vi "Test Sync SMO.vi"() -> ()   [LabVIEW 2019, in "DAQmx.lvclass"]
uses:
  DAQmx.lvclass
  typedefs/DAQmx.Status--enum.ctl
  typedefs/DAQmx.Commands--enum.ctl
  typedefs/DAQ.Config.Timing.Sampling--Cluster.ctl
  typedefs/DAQ.Config.AO--Cluster--Array.ctl
  typedefs/DAQ.Config.AO--Cluster.ctl
  typedefs/DAQ.Config.AO.Range--enum.ctl
  typedefs/DAQ.Config.Device Type--enum.ctl
  typedefs/DAQ.Config.AI--Cluster--Array.ctl
  typedefs/DAQ.Config.AI--Cluster.ctl
  typedefs/DAQ.Config.AI.Coupling--enum.ctl
  typedefs/DAQ.Config.AI.Range--enum.ctl
  C:/Program Files/National Instruments/LabVIEW 2019/vi.lib/JKI/JKI SMO/SMO/SMO.lvclass
  <vilib>/JKI/JKI SMO/SMO/SMO.lvclass/SMO.ctl
  <vilib>/JKI/JKI SMO/SMO/Typedefs/SMOState --Enum.ctl
  typedefs/DAQ.Config.Timing--Cluster.ctl
  DAQmx.lvclass/DAQmx.ctl
  6507ff78-a65c-40b2-afe2-716dbe4badb2.vi
  <vilib>/JKI/JKI SMO/SMO/Private/ReftoDVR--SMO.vi
  <vilib>/JKI/JKI SMO/SMO/SMO.lvclass
panel:
  out "delimited string":string
  out "Generator create":i32=5
  out "Generator 'timeout'":i32=729
  out "Generator":i32=733
  out "Waveform Chart":i32(graph)
  out "Waveform Graph":waveform(dbl)[](graph)
  in  "AIconfig":T1=[{"Channels"="PXI1Slot3/ai0", "Coupling"=10050, "Range"=enum."±0.316", "input terminal configuration"=-1, "Type"=enum."PXI-446x"}, {"Channels"="PXI1Slot3/ai1", "Coupling"=10050, "Range"=enum."±0.316", "input terminal configuration"=-1, "Type"=enum."PXI-446x"}, {"Channels"="PXI1Slot5/ai0", "Coupling"=10050, "Range"=enum."±0.316", "input terminal configuration"=-1, "Type"=enum."PXI-446x"}, {"Channels"="PXI1Slot5/ai1", "Coupling"=10050, "Range"=enum."±0.316", "input terminal configuration"=-1, "Type"=enum."PXI-446x"}, {"Channels"="PXI1Slot6/ai0", "Coupling"=10050, "Range"=enum."±0.316", "input terminal configuration"=-1, "Type"=enum."PXI-446x"}, {"Channels"="PXI1Slot6/ai1", "Coupling"=10050, "Range"=enum."±0.316", "input terminal configuration"=-1, "Type"=enum."PXI-446x"}, {"Channels"="PXI1Slot7/ai0", "Coupling"=10050, "Range"=enum."±0.316", "input terminal configuration"=-1, "Type"=enum."PXI-446x"}, {"Channels"="PXI1Slot7/ai1", "Coupling"=10050, "Range"=enum."±0.316", "input terminal configuration"=-1, "Type"=enum."PXI-446x"}, {"Channels"="PXI1Slot8/ai0", "Coupling"=10050, "Range"=enum."±0.316", "input terminal configuration"=-1, "Type"=enum."PXI-446x"}, {"Channels"="PXI1Slot8/ai1", "Coupling"=10050, "Range"=enum."±0.316", "input terminal configuration"=-1, "Type"=enum."PXI-446x"}] {"input terminal configuration" items=[""=-1, "Differential"=10106, "Pseudodifferential"=12529]; "Coupling" items=[""=0, "AC"=10045, "DC"=10050, "GND"=10066]}
  in  "AOconfig":T6=[{"Channels"="PXI1Slot3/ao0", "Range"=enum."±0.1", "output terminal configuration"=-1, "Type"=enum."PXI-446x"}, {"Channels"="PXI1Slot3/ao1", "Range"=enum."±0.1", "output terminal configuration"=-1, "Type"=enum."PXI-446x"}, {"Channels"="PXI1Slot5/ao0", "Range"=enum."±0.1", "output terminal configuration"=-1, "Type"=enum."PXI-446x"}, {"Channels"="PXI1Slot5/ao1", "Range"=enum."±0.1", "output terminal configuration"=-1, "Type"=enum."PXI-446x"}, {"Channels"="PXI1Slot6/ao0", "Range"=enum."±0.1", "output terminal configuration"=-1, "Type"=enum."PXI-446x"}, {"Channels"="PXI1Slot6/ao1", "Range"=enum."±0.1", "output terminal configuration"=-1, "Type"=enum."PXI-446x"}, {"Channels"="PXI1Slot7/ao0", "Range"=enum."±0.1", "output terminal configuration"=-1, "Type"=enum."PXI-446x"}, {"Channels"="PXI1Slot7/ao1", "Range"=enum."±0.1", "output terminal configuration"=-1, "Type"=enum."PXI-446x"}, {"Channels"="PXI1Slot8/ao0", "Range"=enum."±0.1", "output terminal configuration"=-1, "Type"=enum."PXI-446x"}, {"Channels"="PXI1Slot8/ao1", "Range"=enum."±0.1", "output terminal configuration"=-1, "Type"=enum."PXI-446x"}] {"output terminal configuration" items=[""=-1, "Differential"=10106, "Pseudodifferential"=12529]}
  in  "setAIconfig":bool
  in  "setAOconfig":bool
  in  "setTiming":bool
  in  "Sampling":T9={"Fs"=1000.0, "#s"=128} {"Fs" format="%#_13g"}
  in  "setState":bool
  in  "State":T10=enum."auto"
  out "Status":T11
  out "error out":errorcluster
  # "Close Panel to stop the SMO\n(press the \"X\")"
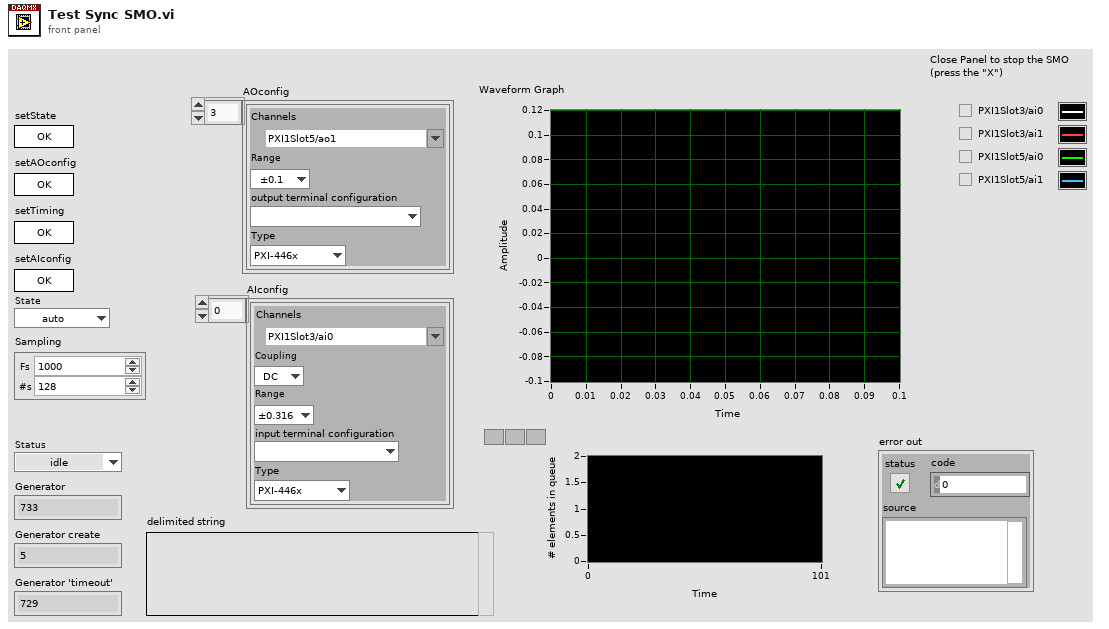
[diagram p1: front panel]
types:
  T1 = typedef "DAQmx.lvclass/DAQ.Config.AI--Cluster--Array.ctl" = T2[]
  T2 = typedef "DAQmx.lvclass/DAQ.Config.AI--Cluster.ctl" = cluster{"Channels":tag, "Coupling":T3, "Range":T4, "input terminal configuration":i32, "Type":T5}
  T3 = typedef "DAQmx.lvclass/DAQ.Config.AI.Coupling--enum.ctl" = u16
  T4 = typedef "DAQmx.lvclass/DAQ.Config.AI.Range--enum.ctl" = enum16{"±0.316", "±1.00", "±3.16", "±10.0", "±31.6", "±42.4", ""}
  T5 = typedef "DAQmx.lvclass/DAQ.Config.Device Type--enum.ctl" = enum16{"None", "USB-4431", "PXI-446x"}
  T6 = typedef "DAQmx.lvclass/DAQ.Config.AO--Cluster--Array.ctl" = T7[]
  T7 = typedef "DAQmx.lvclass/DAQ.Config.AO--Cluster.ctl" = cluster{"Channels":tag, "Range":T8, "output terminal configuration":i32, "Type":T5}
  T8 = typedef "DAQmx.lvclass/DAQ.Config.AO.Range--enum.ctl" = enum16{"±0.1", "±1.0", "±3.5", "±10.0", ""}
  T9 = typedef "DAQmx.lvclass/DAQ.Config.Timing.Sampling--Cluster.ctl" = cluster{"Fs":dbl, "#s":i32}
  T10 = typedef "DAQmx.lvclass/DAQmx.Commands--enum.ctl" = enum16{"idle", "start", "stop", "calibrate", "auto", "exit"}
  T11 = typedef "DAQmx.lvclass/DAQmx.Status--enum.ctl" = enum16{"idle", "calibrating", "configuring", "creating", "created", "starting", "started", "stopping", "stopped", "clearing", "error"}
  T12 = typedef "SMO.lvclass/Public Events.ctl" = cluster{"Error":refnum<user-event>, "State":refnum<user-event>, "Reserve State":refnum<user-event>}
  T13 = typedef "DAQmx.lvclass/PublicEvents--Cluster.ctl" = cluster{"Status":refnum<user-event>, "Devices":refnum<user-event>, "Calibration":refnum<user-event>, "Sampling":refnum<user-event>, "AOconfig":refnum<user-event>, "AIconfig":refnum<user-event>, "Waveforms":refnum<user-event>}
  T14 = cluster{"Event Registration Refnum":refnum<event-registration>}
  T15 = typedef "SMO.lvclass/SMOState --Enum.ctl" = enum16{"unknown", "Created", "Started", "Stopped"}
  T16 = typedef "DAQmx.lvclass/DAQ.Config.Timing--Cluster.ctl" = cluster{"Sampling":T9, "Fs_Out":dbl}
  T17 = typedef "DAQmx.lvclass/DeviceInfo--Cluster.ctl" = cluster{"DeviceName":string, "DevIsSimulated":bool, "DeviceSerialNumber":string, "ProductType":string, "ProductCategory":i32, "ProductNumber":u32, "ChassisNumber":u32, "SlotNumber":u32, "ChassisName":string, "ChassisSerialNumber":string, "DevTemp":dbl, "SelfCal.LastDate/Time":string, "SelfCal.LastTemp":dbl, "calibration due?":bool}
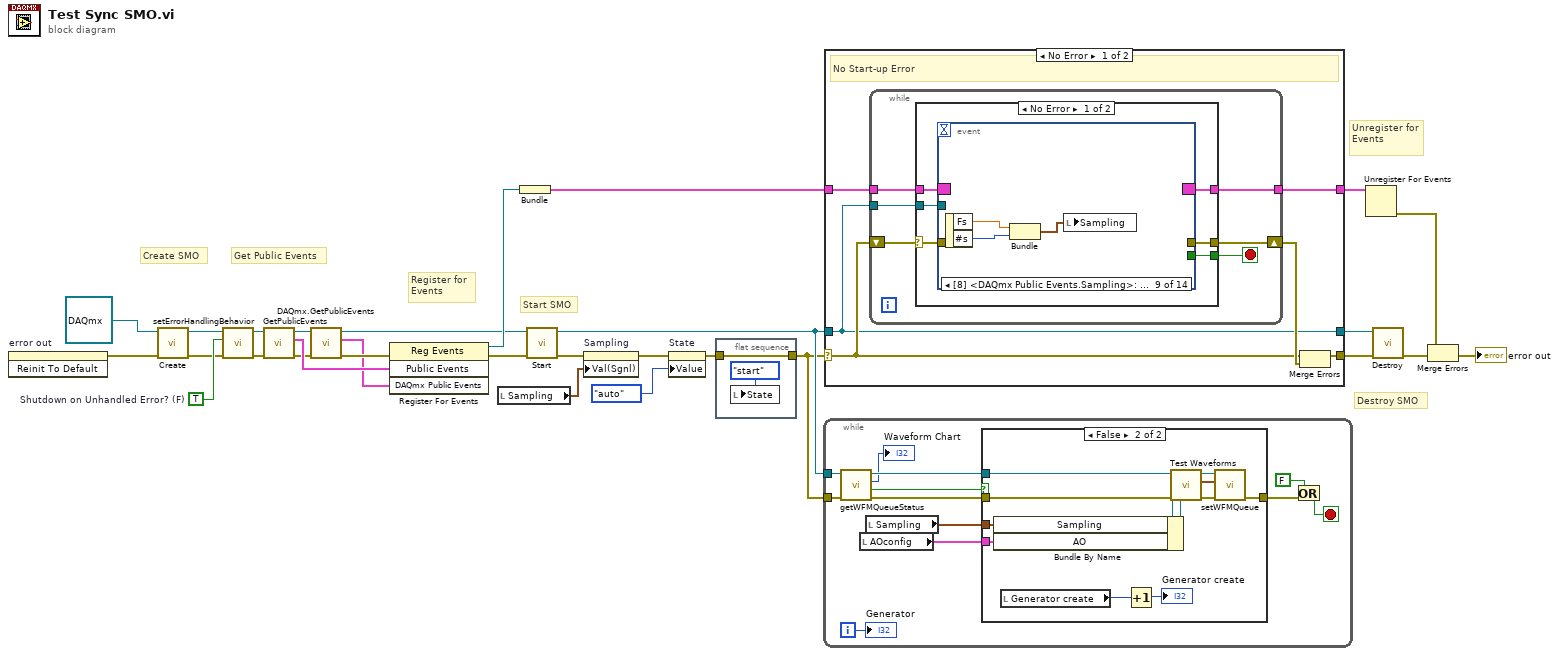
[diagram p0: block diagram]
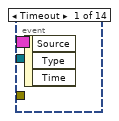
[diagram p2: hidden frame]
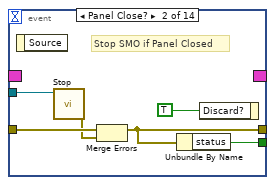
[diagram p3: hidden frame]
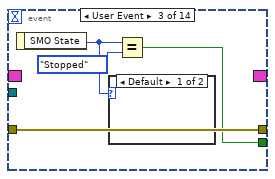
[diagram p4: hidden frame]
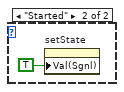
[diagram p5: hidden frame]
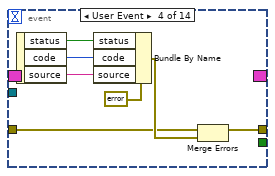
[diagram p6: hidden frame]
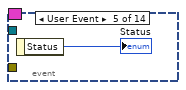
[diagram p7: hidden frame]
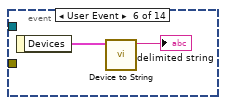
[diagram p8: hidden frame]
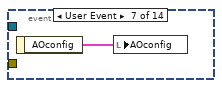
[diagram p9: hidden frame]
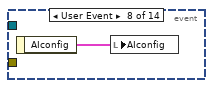
[diagram p10: hidden frame]
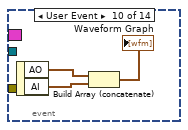
[diagram p11: hidden frame]
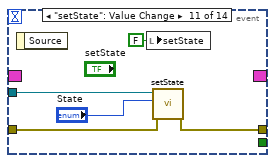
[diagram p12: hidden frame]
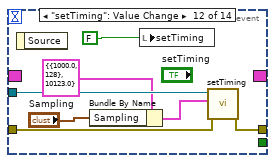
[diagram p13: hidden frame]
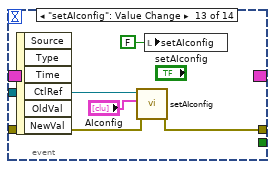
[diagram p14: hidden frame]
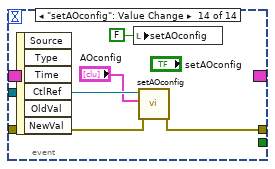
[diagram p15: hidden frame]
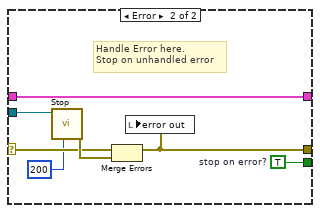
[diagram p16: hidden frame]
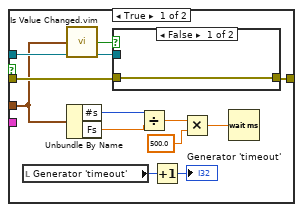
[diagram p18: hidden frame]
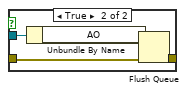
[diagram p19: hidden frame]
diagram:
  w27 = TRUE  # Shutdown on Unhandled Error? (F)
  # "Get Public Events"
  # "Start SMO"
  # "Destroy SMO"
  # "Create SMO"
  # "Unregister for Events"
  # "Register for Events"
  n1 = invoke on="error out" class="Clust (strict)" method="Reinit To Default"() -> (error out=w28:errorcluster)  [unwired: 3 in, 2 out]
  n2 = call <vilib>:"Create.vi"("error in (no error)"=w28, "SMO"=refnum<class "DAQmx.lvclass"> refnum ("DAQmx.lvclass")) -> ("error out"=w25:errorcluster, "SMO out"=w23:refnum<class "DAQmx.lvclass">)  [unwired: 7 in, 1 out]
  n3 = call <vilib>:"setErrorHandlingBehavior.vi"("error in (no error)"=w25, "Shutdown on Unhandled Error? (F)"=w27, "SMO in"=w23) -> ("error out"=w26:errorcluster, "SMO out"=w24:refnum<class "DAQmx.lvclass">)  [unwired: 7 in]
  n4 = call <vilib>:"GetPublicEvents.vi"("error in (no error)"=w26, "SMO"=w24) -> ("error out"=w12:errorcluster, "Public Events"=w21:T12, "SMO out"=w9:refnum<class "DAQmx.lvclass">)  [unwired: 7 in]
  n5 = call "DAQmx.GetPublicEvents.vi"("error in (no error)"=w12, "DAQmx"=w9) -> ("error out"=w11:errorcluster, "DAQmx Public Events"=w10:T13, "DAQmx out"=w8:refnum<class "DAQmx.lvclass">)  [unwired: 7 in]
  n6 = register-events(error in=w11, w21, w10) -> (reference out=w19:refnum<event-registration>, error out=w20:errorcluster)  [unwired: 1 in]
  n7 = local read "Sampling"() -> (w1:T9)
  n8 = Bundle("Event Registration Refnum"=w19) -> (w15:T14)  [unwired: 1 in]
  n9 = call <vilib>:"Start.vi"("error in (no error)"=w20, "SMO"=w8) -> ("error out"=w6:errorcluster, "SMO out"=w7:refnum<class "DAQmx.lvclass">)  [unwired: 8 in]
  n10 = property on="Sampling" class="Clust (strict)"(error in=w6, "Val(Sgnl)"=w1) -> (error out=w5:errorcluster)  [unwired: 1 in, 1 out]
  n11 = property on="State" class="Enum (strict)"(error in=w5, "Value"=DAQmx.Commands--enum."auto" ("Value (Signaling)")) -> (error out=w2:errorcluster)  [unwired: 1 in, 1 out]
  n12 = flat-sequence {
    tunnel: [w31] -> w3
    tunnel: w2 -> [w31]
    frame #0 {
      n13 = local write "State"(DAQmx.Commands--enum."start" ("Value (Signaling)")) -> ()
    }
  }
  n14 = while {
    tunnel: w7 -> [w40]
    tunnel: w3 -> [w36]
    i -> [w43]
    stop <- w42 stop-if-true
    n15 = call "getWFMQueueStatus.vi"("error in (no error)"=w36, "DAQmx in"=w40) -> ("error out"=w39:errorcluster, "Min AO Queue Filled"=w33:bool, "AO queue #"=→"Waveform Chart":i32, "DAQmx out"=w41:refnum<class "DAQmx.lvclass">)  [unwired: 6 in]
    n16 = local read "AOconfig"() -> (w34:T6)
    n17 = local read "Sampling"() -> (w35:T9)
    n18 = case shown="False" w33 {
      tunnel: w41 -> [w48 w64]
      tunnel: w39 -> [w47 w67]
      tunnel: [w46 w65] -> w38
      tunnel: w35 -> [w44 w61]
      tunnel: w34 -> [_ w62]
      frame True {
        n19 = local read "Generator 'timeout'"() -> (w55:i32)
        n20 = call "Is Value Changed.vim"("value"=w44) -> ("changed or first call?"=w45:bool)
        n21 = Unbundle By Name(w44) -> ("#s"=w50:i32, "Fs"=w49:dbl)
        n22 = case shown="False" w45 {
          tunnel: w48 -> [_ w60]
          tunnel: w47 -> [w56 w58]
          tunnel: [w56 w57] -> w46
          frame False {
          }
          frame True {
            n23 = Unbundle By Name(w60) -> ("AO"=w59:refnum<queue>)
            n24 = Flush Queue(queue=w59, error in (no error)=w58) -> (error out=w57:errorcluster)  [unwired: 2 out]
          }
        }
        n25 = Divide(x=w50, y=w49) -> (x/y=w53:dbl)
        n26 = Increment(x=w55) -> (x+1=→"Generator 'timeout'":i32)
        n27 = Multiply(x=w53, y=500.0) -> (x*y=w52:dbl)
        n28 = Wait (ms)(milliseconds to wait=w52) -> ()  [unwired: 1 out]
      }
      frame False {
        n29 = Bundle By Name(cluster=w64, "Sampling"=w61, "AO"=w62) -> (w63:refnum<class "DAQmx.lvclass">)
        n30 = local read "Generator create"() -> (w70:i32)
        n31 = Increment(x=w70) -> (x+1=→"Generator create":i32)
        n32 = call "Test Waveforms.vi"("error in (no error)"=w67, "DAQmx in"=w63) -> ("error out"=w66:errorcluster, "Waveforms"=w68:waveform(dbl)[], "DAQmx out"=w69:refnum<class "DAQmx.lvclass">)  [unwired: 7 in]
        n33 = call "setWFMQueue.vi"("error in (no error)"=w66, "AO"=w68, "DAQmx in"=w69) -> ("error out"=w65:errorcluster)  [unwired: 7 in, 1 out]
      }
    }
    n34 = Or(x=FALSE, y=w38) -> (x .or. y?=w42:bool)
    "Generator" <- w43
  }
  n35 = case shown="No Error" w3 {
    selector: w3 -> [w73 w149]
    tunnel: [w77 w150] -> w14
    tunnel: w15 -> [w76 w150]
    tunnel: [w74 w149] -> w22
    tunnel: w7 -> [w72 w148]
    tunnel: [w72 w148] -> w29
    frame No Error {
      # "No Start-up Error"
      n36 = while {
        shift-right: [w82] -> w75
        shift-left: w73 -> [w78]
        tunnel: w76 -> [w81]
        tunnel: [w80] -> w77
        tunnel: w72 -> [w79]
        stop <- w83 stop-if-true
        n37 = case shown="No Error" w78 {
          selector: w78 -> [w84 w144]
          tunnel: [w89 w147] -> w83
          tunnel: [w88 w141] -> w82
          tunnel: w81 -> [w87 w146]
          tunnel: [w86 w146] -> w80
          tunnel: w79 -> [w85 w143]
          frame No Error {
            n38 = event shown="[8] <DAQmx Public Events.Sampling>: User Event" {
              selector: w87 -> [_ _ _ _ _ _ _ _ _ _ _ _ _ _]
              dyn-events: [_ _ _ _ _ _ _ _ _ _ _ _ _ _] -> w86
              timeout: _ -> [_ _ _ _ _ _ _ _ _ _ _ _ _ _]
              tunnel: [_ w93 w97 _ _ _ _ _ _ _ _ _ _ _] -> w89
              tunnel: w85 -> [_ w95 _ _ _ _ _ _ _ _ w122 w130 w135 w140]
              tunnel: [_ w90 w98 w101 _ _ _ _ _ _ w121 w129 w132 w138] -> w88
              tunnel: w84 -> [_ w92 w98 w102 _ _ _ _ _ _ w120 w128 w133 w139]
              event Timeout {
                n39 = event-data() -> ()  [unwired: 1 in, 3 out]
              }
              event Panel Close? {
                # "Stop SMO if Panel Closed"
                n40 = event-data() -> ()  [unwired: 1 in, 1 out]
                n41 = call <vilib>:"Stop.vi"("SMO"=w95) -> ("error out"=w91:errorcluster)  [unwired: 9 in, 1 out]
                n42 = Merge Errors(w92, w91) -> (w90:errorcluster)
                n43 = Unbundle By Name(w90) -> ("status"=w93:bool)
                n44 = event-data("Discard?"=TRUE ("OK")) -> ()  [unwired: 1 in, 1 out]
              }
              event User Event {
                n45 = event-data() -> ("SMO State"=w96:T15)  [unwired: 1 in]
                n46 = case shown="Default" w96 {
                  frame Default {
                  }
                  frame "Started" {
                    n47 = property on="setState" class="Bool (strict)"("Val(Sgnl)"=TRUE) -> ()  [unwired: 2 in, 2 out]
                  }
                }
                n48 = Equal?(x=w96, y=SMOState_--Enum."Stopped") -> (x = y?=w97:bool)
              }
              event User Event {
                n49 = event-data() -> ("status"=w107:bool, "code"=w106:i32, "source"=w105:string)  [unwired: 1 in]
                n50 = Bundle By Name(cluster=errorcluster {"status"=FALSE, "code"=0, "source"=""} ("error out"), "status"=w107, "code"=w106, "source"=w105) -> (w103:errorcluster)
                n51 = Merge Errors(w102, w103) -> (w101:errorcluster)
              }
              event User Event {
                n52 = event-data() -> ("Status"=→"Status":T11)  [unwired: 1 in]
              }
              event User Event {
                n53 = event-data() -> ("Devices"=w110:T17[])  [unwired: 1 in]
                n54 = call "Device to String.vi"("Devices"=w110) -> ("delimited string"=→"delimited string":string)  [unwired: 10 in]
              }
              event User Event {
                n55 = event-data() -> ("AOconfig"=w111:T6)  [unwired: 1 in]
                n56 = local write "AOconfig"(w111) -> ()
              }
              event User Event {
                n57 = event-data() -> ("AIconfig"=w112:T1)  [unwired: 1 in]
                n58 = local write "AIconfig"(w112) -> ()
              }
              event User Event {
                n59 = event-data() -> ("Fs"=w113:dbl, "#s"=w114:i32)  [unwired: 1 in]
                n60 = Bundle("Fs"=w113, "#s"=w114) -> (w115:cluster{"Fs":dbl, "#s":i32})  [unwired: 1 in]
                n61 = local write "Sampling"(w115) -> ()
              }
              event User Event {
                n62 = event-data() -> ("AO"=w116:waveform(dbl)[], "AI"=w117:waveform(dbl)[])  [unwired: 1 in]
                n63 = Build Array (concatenate)(w116, w117) -> (→"Waveform Graph":waveform(dbl)[])
              }
              event "setState": Value Change {
                n64 = event-data() -> ()  [unwired: 1 in, 1 out]
                n65 = local write "setState"(FALSE ("setState")) -> ()
                n66 = call "setState.vi"("error in (no error)"=w120, "Command"="State", "DAQmx in"=w122) -> ("error out"=w121:errorcluster)  [unwired: 7 in, 1 out]
              }
              event "setTiming": Value Change {
                n67 = event-data() -> ()  [unwired: 1 in, 1 out]
                n68 = Bundle By Name(cluster=T16 {"Sampling"={"Fs"=1000.0, "#s"=128}, "Fs_Out"=10123.0} ("Timing"), "Sampling"="Sampling") -> (w124:T16)
                n69 = local write "setTiming"(FALSE ("setTiming")) -> ()
                n70 = call "setTiming.vi"("error in (no error)"=w128, "Timing"=w124, "DAQmx in"=w130) -> ("error out"=w129:errorcluster)  [unwired: 7 in, 1 out]
              }
              event "setAIconfig": Value Change {
                n71 = event-data() -> ()  [unwired: 1 in, 6 out]
                n72 = call "setAIconfig.vi"("error in (no error)"=w133, "AIconfig"="AIconfig", "DAQmx in"=w135) -> ("error out"=w132:errorcluster)  [unwired: 7 in, 1 out]
                n73 = local write "setAIconfig"(FALSE ("setAIconfig")) -> ()
              }
              event "setAOconfig": Value Change {
                n74 = event-data() -> ()  [unwired: 1 in, 6 out]
                n75 = local write "setAOconfig"(FALSE ("setAOconfig")) -> ()
                n76 = call "setAOconfig.vi"("error in (no error)"=w139, "AOconfig"="AOconfig", "DAQmx in"=w140) -> ("error out"=w138:errorcluster)  [unwired: 7 in, 1 out]
              }
            }
          }
          frame Error {
            w147 = TRUE  # stop on error?
            # "Handle Error here.\nStop on unhandled error"
            n77 = call <vilib>:"Stop.vi"("timeout in ms (-1)"=200, "SMO"=w143) -> ("error out"=w145:errorcluster)  [unwired: 8 in, 1 out]
            n78 = Merge Errors(w144, w145) -> (w141:errorcluster)
            n79 = local write "error out"(w141) -> ()
          }
        }
      }
      n80 = Merge Errors(w73, w75) -> (w74:errorcluster)
    }
    frame Error {
      # "Error occured before starting the process"
    }
  }
  n81 = Unregister For Events(event registration refnum=w14) -> (error out=w16:errorcluster)  [unwired: 1 in]
  n82 = call <vilib>:"Destroy.vi"("error in (no error)"=w22, "SMO"=w29) -> ("error out"=w18:errorcluster)  [unwired: 9 in]
  n83 = Merge Errors(w16, w18) -> (→"error out":errorcluster)
